vi "List Files.vi"(8 "error in (no error)":errorcluster, 11 "CSM-Static-Variable-Manager in":refnum<class "CSM-Static-Variable-Manager.lvclass">) -> (0 "error out":errorcluster, 1 "File List":path[](array[path]), 3 "CSM-Static-Variable-Manager out":refnum<class "CSM-Static-Variable-Manager.lvclass">)   [LabVIEW 2017, in "INI-Static-Variable-Support.lvlib" / "CSM-Static-Variable-Manager.lvclass"]
uses:
  CSM-Static-Variable-Manager.lvclass
  CSM-Static-Variable-Manager.lvclass/CSM-Static-Variable-Manager.ctl
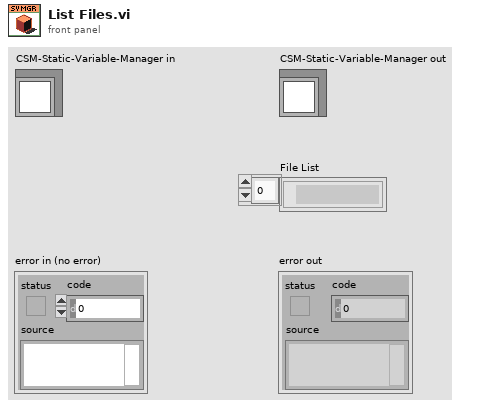
[diagram p1: front panel]
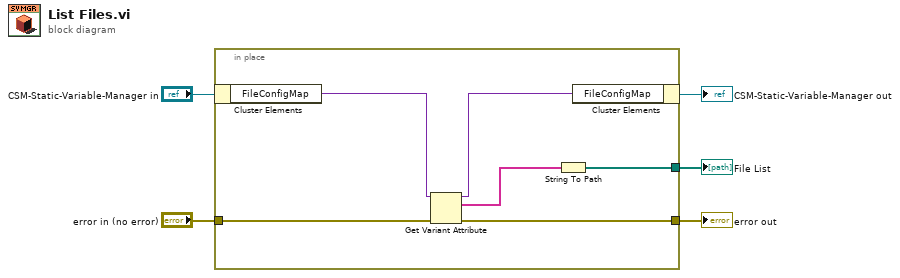
[diagram p0: block diagram]
diagram:
  n1 = in-place {
    in-place-border: "error in (no error)" -> [w11]
    in-place-border: [w10] -> w2
    in-place-border: [w6] -> w1
    n2 = in-place-cluster #1("CSM-Static-Variable-Manager in") -> ("FileConfigMap"=w9:variant)
    n3 = Get Variant Attribute(Variant=w9, error in=w11) -> (duplicate Variant=w8:variant, names=w7:string[], error out=w10:errorcluster)  [unwired: 2 in, 1 out]
    n4 = String To Path(string=w7) -> (path=w6:path[])
    n5 = in-place-cluster #1("FileConfigMap"=w8) -> (→"CSM-Static-Variable-Manager out":refnum<class "CSM-Static-Variable-Manager.lvclass">)
  }
  "error out" <- w2
  "File List" <- w1
